vi "ExecuteLV.vi"(8 "error in (no error)":errorcluster, 11 "CallEXEStepBase in":refnum<class "CallEXEStep.lvclass">) -> (0 "error out":errorcluster, 1 "Status":T1, 3 "CallEXEStepBase out":refnum<class "CallEXEStep.lvclass">)   [LabVIEW 2015, in "CallEXEStep.lvclass"]
uses:
  CallEXEStep.lvclass
  Step/STEP_STATUS.ctl
  Step.lvclass
panel:
  out "concatenated string":string
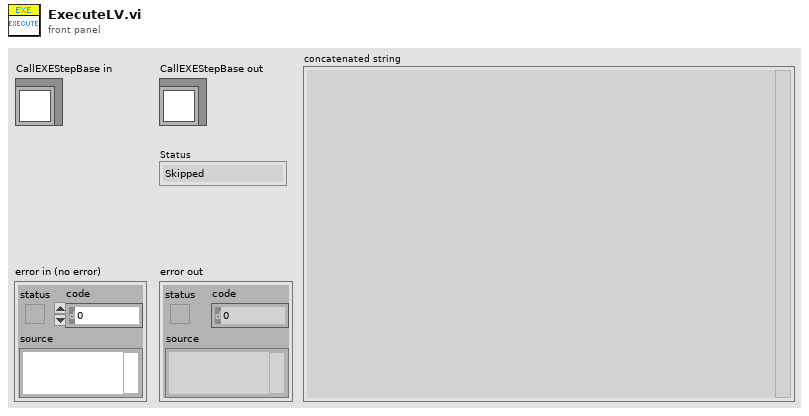
[diagram p1: front panel]
types:
  T1 = typedef "Step.lvclass/STEP_STATUS.ctl" = enum16{"Skipped", "Done", "Passed", "Failed", "Error"}
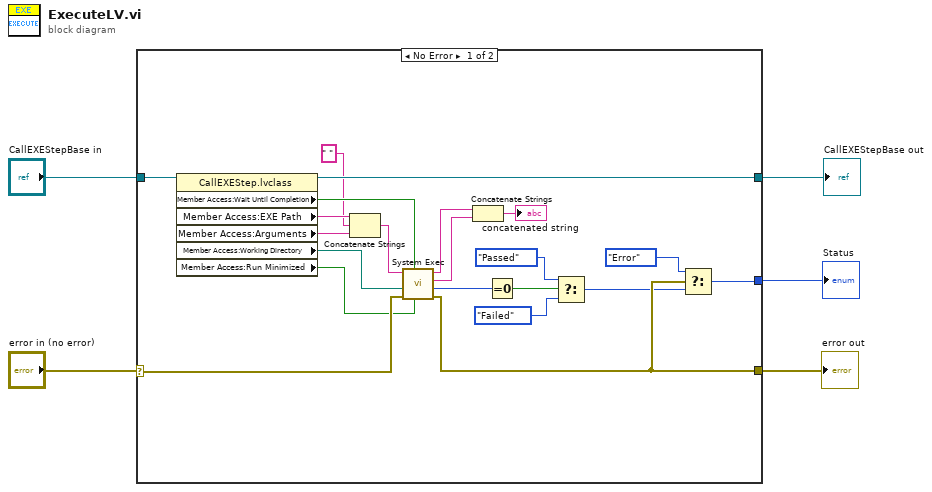
[diagram p0: block diagram]
diagram:
  n1 = case shown="No Error" "error in (no error)" {
    selector: "error in (no error)" -> [w24 w28]
    tunnel: "CallEXEStepBase in" -> [w26 w27]
    tunnel: [w16 w28] -> w3
    tunnel: [w21 w27] -> w2
    tunnel: [w13 _] -> w1
    frame No Error {
      n2 = property class="CallEXEStep.lvclass"(reference=w26) -> (reference out=w21:refnum<class "CallEXEStep.lvclass">, "Member Access:Wait Until Completion"=w25:bool, "Member Access:EXE Path"=w8:string, "Member Access:Arguments"=w9:string, "Member Access:Working Directory"=w23:path, "Member Access:Run Minimized"=w22:bool)  [unwired: 1 in, 1 out]
      n3 = Concatenate Strings(w8, " ", w9) -> (w6:string)
      n4 = call <vilib>:"System Exec.vi"("run minimized? (F)"=w22, "wait until completion? (T)"=w25, "error in (no error)"=w24, "working directory"=w23, "command line"=w6) -> ("error out"=w16:errorcluster, "return code"=w20:i32, "standard error"=w11:string, "standard output"=w12:string)  [unwired: 3 in]
      n5 = Concatenate Strings(w12, w11) -> (→"concatenated string":string)
      n6 = Equal To 0?(x=w20) -> (x = 0?=w19:bool)
      n7 = Select(t=STEP_STATUS."Passed" ("Status"), s=w19, f=STEP_STATUS."Failed" ("Status")) -> (s? t:f=w14:T1)
      n8 = Select(t=STEP_STATUS."Error" ("Status"), s=w16, f=w14) -> (s? t:f=w13:T1)
    }
    frame Error {
    }
  }
  "error out" <- w3
  "CallEXEStepBase out" <- w2
  "Status" <- w1
